vi "Subtract.vi"(10 "A":dbl, 11 "y":dbl) -> (2 "A-y":dbl)   [LabVIEW 2020]
panel:
  in  "Boolean 2":bool
  in  "Boolean":bool
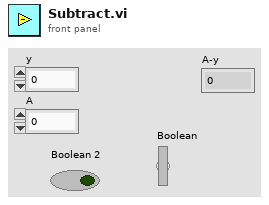
[diagram p1: front panel]
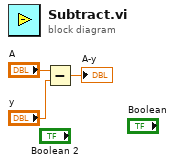
[diagram p0: block diagram]
diagram:
  n1 = Subtract(x="A", y="y") -> (x-y=→"A-y":dbl)
